vi "Characterise Polarisation.vi"() -> ()   [LabVIEW 2019]
panel:
  in  "Background Power (mW)":dbl format="%#_13g"
  in  "?":refnum<k7>(container)
  in  "Wavelength (nm)":dbl=400.0 caption="Wavelength (0.0)"
  in  "?":T1(tab)
  out "?":cluster{dbl[], dbl[]}[](graph)
  out "Current Scan Angle:":i32
  in  "Step Size:":i32=5
  in  "Full Rotation":bool
  in  "?":bool
  out "Stokes Vector:":dbl[](array[numeric]) format="%.3g"
  out "XY Graph 2":cluster{dbl[], dbl[]}[](graph)
  in  "?":refnum<k7>(container)
  out "Zero Angle on Stage :":dbl format="%#.1g"
  in  "?":enum32{"First Waveplate", "Second Waveplate"}(tab)
  out "XY Graph":cluster{dbl[], dbl[]}[](graph)
  out "?":cluster{dbl[], dbl[]}[](graph)
  out "?":cluster{dbl[], dbl[]}[](graph)
  out "Stokes Vector 2":dbl[](array[numeric]) format="%.3g"
  out "CPL 1:":dbl format="%#_4g"
  out "Stokes Vector":dbl[](array[numeric]) format="%.3g"
  out "CPL 2:":dbl format="%#.2g"
  in  "Full":bool
  in  "Step Size:":i32=10
  out "?":i32
  out "Current Scan Angle:":i32
  in  "?":bool
  in  "?":bool
  # "Polarisation Characterisation"
  # "This software uses the rotation of a quarter-wave plate and a power meter to characterise any given input laser polarisation. Specifically, it has been designed to produce and characterise right and left circulalry polarised light by using a motorised rotating waveplate.\n\nBefore use, please ensure:\n\n     - the power meter is turned on and connected to the PC/Laptop\n     using the mini-USB cable\n\n     - the motorised waveplate (if using) is connected to the \n     PC/Laptop using the USB 3.0 cable\n\n     - the laser beam is aimed at the power meter\n\n     - a polariser is placed in the beam path before the power meter\n\n     - the correct operating wavelength has been entered below\n     (the default is 400 nm)\n\nThen select the required function from the tab list, complete any further necessary steps and press 'Run' to execute the code."
  # "Half Rotation"
  # "This tab is used to calculate the Stoke's vector for any given input polarisation.\n\n     1. Choose to perform the measurment over a full or half rotation of the waveplate. The default is a full rotation.\n\n     2. Set the 'Step Size' for the quarter-wave plate. This must be an even divisor of 180. The default value is 10. \n\n     3. Insert the quarter-wave plate into the beam path before the polariser. Set the waveplate to zero degrees.\n\n     4. 'Run' the code.\n\n     5. Set the waveplate to the 'Current Scan Angle' and press 'Record' to save the power meter reading. Repeat this for all scan angles.\n\n     6. The scan will be displayed on the graph along with a fit using various sines and cosines (see paper for details). The Stokes vector will be displayed adjacent."
  # "This tab is used to produce pure circularly polarised light.\n\n     1. Set the perameters for the Stokes vector measurment.\n\n     2. 'Run' the code. This will find the two CPL angles on the waveplate.\n\n     3. Set the second waveplate to the 'Current Scan Angle' and press record. Repeat for poth angles.\n\n     4. The CPL angles and associated Stokes vectors are calculated and shown adjacent."
  # "Half"
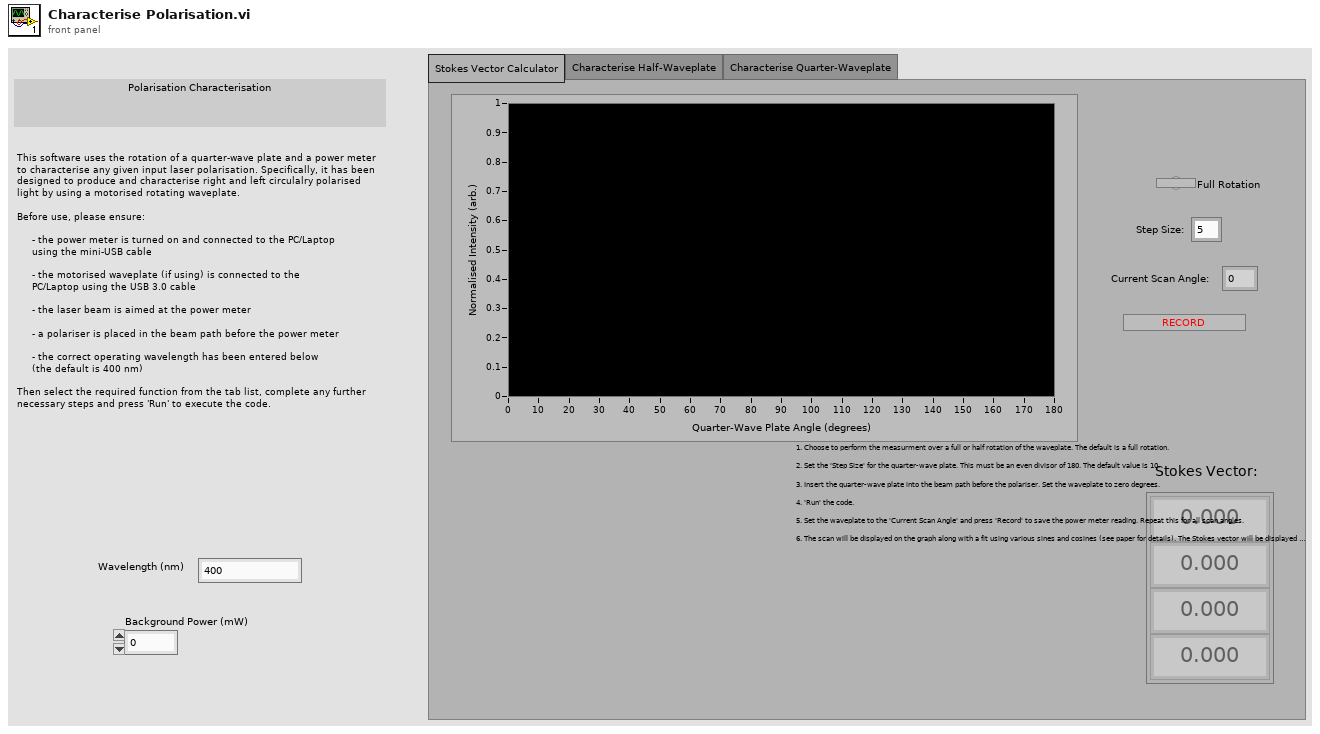
[diagram p1: front panel]
types:
  T1 = enum32{"Stokes Vector Calculator", "Characterise Half-Waveplate", "Characterise Quarter-Waveplate"}
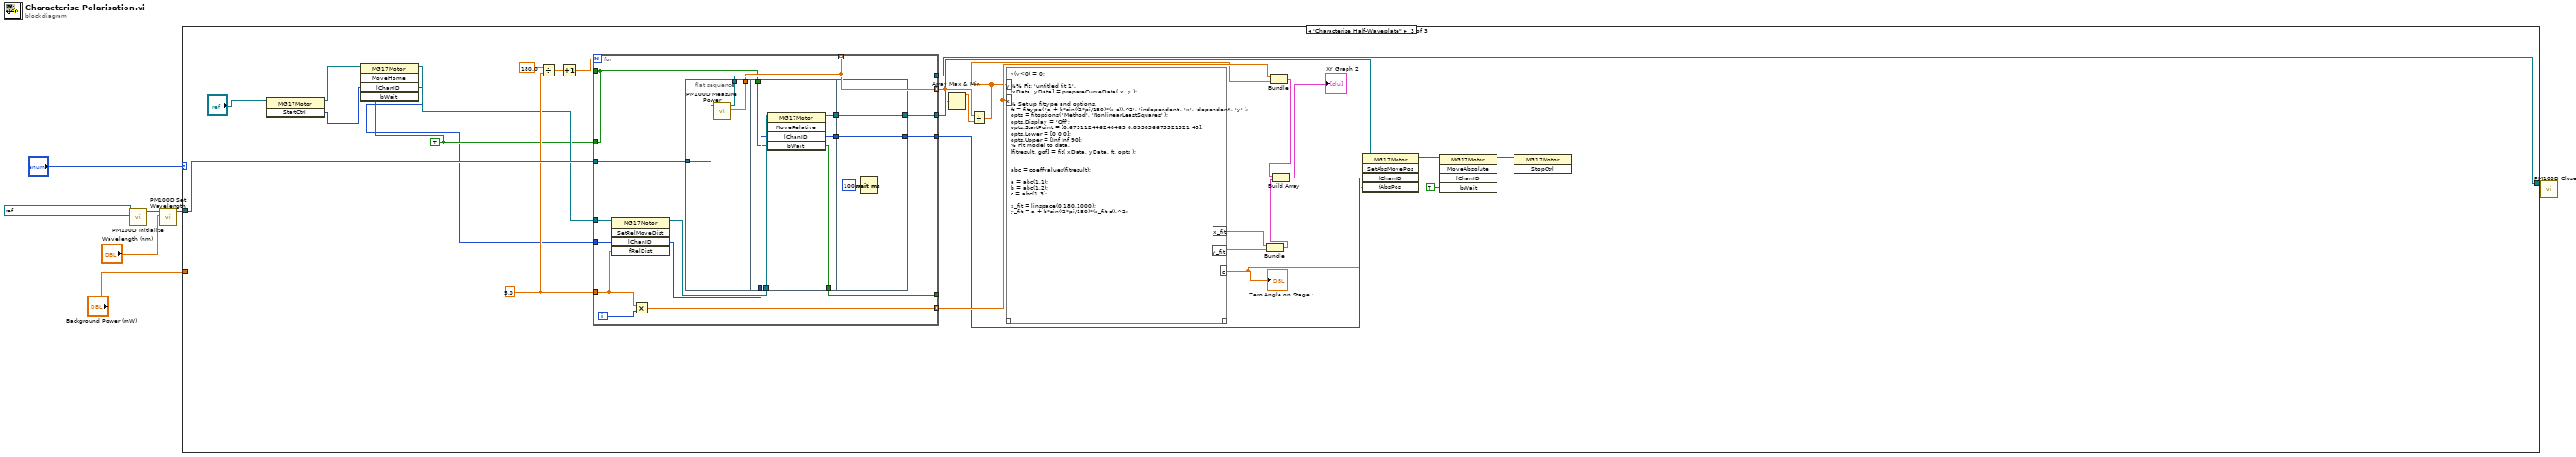
[diagram p0: block diagram]
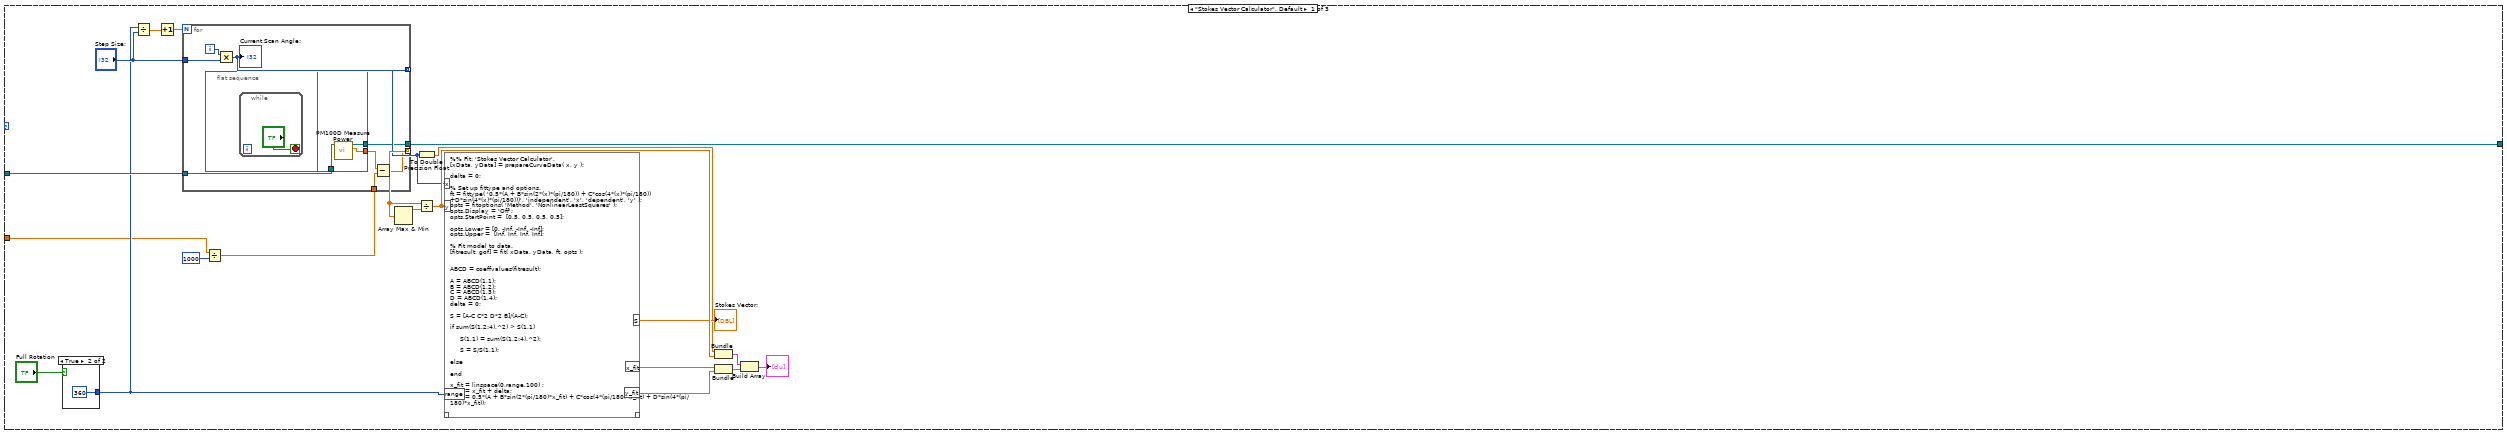
[diagram p2: hidden frame]
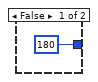
[diagram p3: hidden frame]
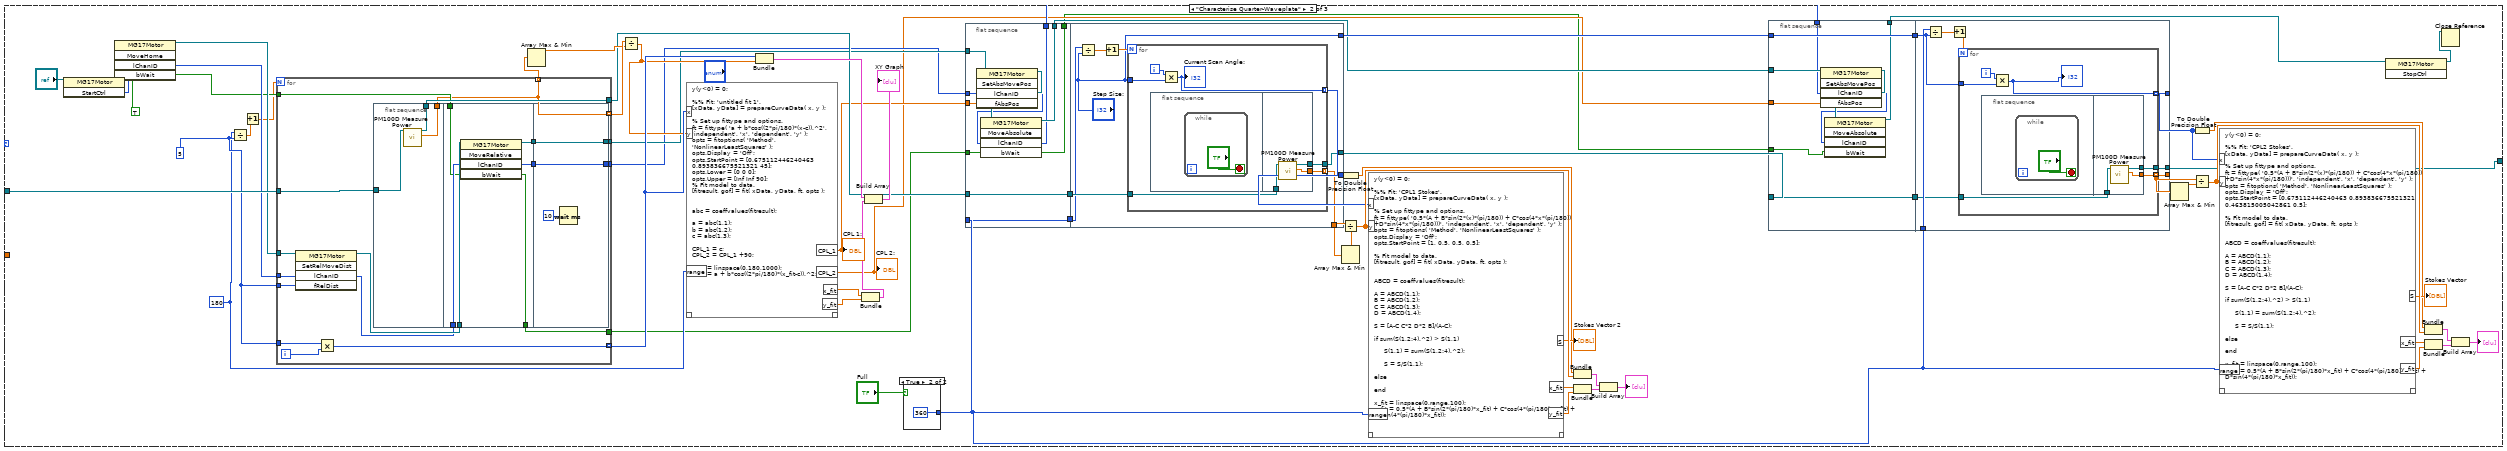
[diagram p4: hidden frame]
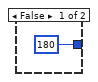
[diagram p5: hidden frame]
diagram:
  n1 = call <instrlib>:"PM100D Initialize.vi"("resource name"=refnum<visa-resource-name> "USB0::0x1313::0x8079::P1002885::INSTR") -> ("instrument handle out"=w6:refnum<visa-resource-name>)  [unwired: 9 in, 1 out]
  n2 = call <instrlib>:"PM100D Set Wavelength.vi"("Wavelength (0.0)"="Wavelength (nm)", "instrument handle"=w6) -> ("instrument handle out"=w3:refnum<visa-resource-name>)  [unwired: 8 in, 1 out]
  n3 = case shown="\"Characterise Half-Waveplate\"" "?" {
    tunnel: w3 -> [w25 w102 w220]
    tunnel: [w23 w57 w214] -> w2
    tunnel: "Background Power (mW)" -> [w10 _ _]
    frame "Stokes Vector Calculator", Default {
      n4 = case shown="True" "Full Rotation" {
        tunnel: [180 360] -> w11
        frame False {
        }
        frame True {
        }
      }
      n5 = Divide(x=w11, y="Step Size:") -> (x/y=w27:dbl)
      n6 = Increment(x=w27) -> (x+1=w26:dbl)
      n7 = Divide(x=w10, y=1000) -> (x/y=w8:dbl)
      n8 = for {
        N: w26 -> [_]
        tunnel: "Step Size:" -> [w35]
        tunnel: w25 -> [w36]
        tunnel: [w37] -> w14 mode=indexing
        tunnel: [w31] -> w22 mode=indexing
        tunnel: [w34] -> w23
        tunnel: w8 -> [w33]
        i -> [w38]
        n9 = flat-sequence {
          tunnel: w36 -> [w42]
          tunnel: [w41] -> w32
          tunnel: [w40] -> w34
          frame #0 {
            n10 = while {
              stop <- "?" stop-if-true
            }
          }
          frame #1 {
            n11 = call <instrlib>:"PM100D Measure Power.vi"("instrument handle"=w42) -> ("Power"=w41:dbl, "instrument handle out"=w40:refnum<visa-resource-name>)  [unwired: 8 in, 1 out]
          }
        }
        n12 = Multiply(x=w38, y=w35) -> (x*y=w37:i32)
        "Current Scan Angle:" <- w37
        n13 = Subtract(x=w32, y=w33) -> (x-y=w31:dbl)
      }
      n14 = Array Max & Min(array=w22) -> (max value=w21:dbl)  [unwired: 3 out]
      n15 = Divide(x=w22, y=w21) -> (x/y=w20:dbl[])
      n16 = To Double Precision Float(number=w14) -> (double precision float=w13:dbl[])
      n17 = script code="%% Fit: 'Stokes Vector Calculator'.\n[xData, yData] = prepareCurveData( x, y );\n\ndelta = 0;\n\n% Set up fittype and options.\nft = fittype( '0.5*(A + B*sin(2*(x)*(pi/180)) + C*cos(4*(x)*(pi/180)) +D*sin(4*(x)*(pi/180)))', 'independent', 'x', 'dependent', 'y' );\nopts = fitoptions( 'Method', 'NonlinearLeastSquares' );\nopts.Display = 'Off';\nopts.StartPoint =  [0.5, 0.5, 0.5, 0.5];\n\nopts.Lower = [0, -Inf, -Inf, -Inf];\nopts.Upper =  [Inf, Inf, Inf, Inf];\n\n% Fit model to data.\n[fitresult, gof] = fit( xData, yData, ft, opts );\n\n\nABCD = coeffvalues(fitresult);\n\nA = ABCD(1,1); \nB = ABCD(1,2);\nC = ABCD(1,3);\nD = ABCD(1,4);\ndelta = 0;\n\nS = [A-C C*2 D*2 B]/(A-C);\n\nif sum(S(1,2:4).^2) > S(1,1)\n\n     S(1,1) = sum(S(1,2:4).^2);\n\n     S = S/S(1,1);\n\nelse\n\nend\n\nx_fit = linspace(0,range,100) ;\nx_fit = x_fit + delta;\ny_fit = 0.5*(A + B*sin(2*(pi/180)*x_fit) + C*cos(4*(pi/180)*x_fit) + D*sin(4*(pi/180)*x_fit));"("x"=w14, "y"=w20, "range"=w11) -> ("S"=→"Stokes Vector:":dbl[], "x_fit"=w18:dbl[], "y_fit"=w17:dbl[])  [unwired: 1 in, 1 out]
      n18 = Bundle(w13, w20) -> (w16:cluster{dbl[], dbl[]})  [unwired: 1 in]
      n19 = Bundle(w18, w17) -> (w12:cluster{dbl[], dbl[]})  [unwired: 1 in]
      n20 = Build Array(w16, w12) -> (→"?":cluster{dbl[], dbl[]}[])
    }
    frame "Characterise Quarter-Waveplate" {
      w98 = 5 ("Step Size:")
      w89 = 180
      n21 = invoke class="MG17Motor" method="StartCtrl"(reference="?") -> (reference out=w105:refnum<k7>, "StartCtrl"=w103:i32)  [unwired: 2 in, 1 out]
      n22 = invoke class="MG17Motor" method="MoveHome"(reference=w105, "lChanID"=w103, "bWait"=TRUE) -> (reference out=w101:refnum<k7>, "lChanID"=w100:i32, "bWait"=w99:bool)  [unwired: 2 in, 2 out]
      n23 = Divide(x=w89, y=w98) -> (x/y=w97:dbl)
      n24 = Increment(x=w97) -> (x+1=w96:dbl)
      n25 = for {
        N: w96 -> [_]
        tunnel: w102 -> [w181]
        tunnel: w101 -> [w180]
        tunnel: w100 -> [w179]
        tunnel: w98 -> [w178]
        tunnel: [w177] -> w71
        tunnel: [w169] -> w87 mode=indexing
        tunnel: w99 -> [w174]
        tunnel: w98 -> [w172]
        tunnel: [w171] -> w95 mode=indexing
        tunnel: [w170] -> w53
        tunnel: [w169] -> w88 mode=indexing
        tunnel: [w168] -> w52
        tunnel: [w167] -> w50
        i -> [w173]
        n26 = invoke class="MG17Motor" method="SetRelMoveDist"(reference=w180, "lChanID"=w179, "fRelDist"=w178) -> (reference out=w176:refnum<k7>, "lChanID"=w175:i32)  [unwired: 2 in, 3 out]
        n27 = Multiply(x=w172, y=w173) -> (x*y=w171:i32)
        n28 = flat-sequence {
          tunnel: w181 -> [w184]
          tunnel: [w183] -> w177
          tunnel: [w182] -> w169
          tunnel: w176 -> [w190]
          tunnel: w175 -> [w189]
          tunnel: w174 -> [w188]
          tunnel: [w185] -> w167
          tunnel: [w187] -> w166
          tunnel: [w186] -> w165
          tunnel: [w192] -> w168
          tunnel: [w193] -> w170
          tunnel: w166 -> [w193]
          tunnel: w165 -> [w192]
          frame #0 {
            n29 = call <instrlib>:"PM100D Measure Power.vi"("instrument handle"=w184) -> ("Power"=w182:dbl, "instrument handle out"=w183:refnum<visa-resource-name>)  [unwired: 8 in, 1 out]
          }
          frame #1 {
            n30 = invoke class="MG17Motor" method="MoveRelative"(reference=w190, "lChanID"=w189, "bWait"=w188) -> (reference out=w187:refnum<k7>, "lChanID"=w186:i32, "bWait"=w185:bool)  [unwired: 2 in, 2 out]
          }
          frame #2 {
            n31 = Wait (ms)(milliseconds to wait=u32 10) -> ()  [unwired: 1 out]
          }
        }
      }
      n32 = Array Max & Min(array=w88) -> (max value=w86:dbl)  [unwired: 3 out]
      n33 = Divide(x=w87, y=w86) -> (x/y=w85:dbl[])
      n34 = script code="y(y<0) = 0;\n\n%% Fit: 'untitled fit 1'.\n[xData, yData] = prepareCurveData( x, y );\n\n% Set up fittype and options.\nft = fittype( 'a + b*cos((2*pi/180)*(x-c)).^2', 'independent', 'x', 'dependent', 'y' );\nopts = fitoptions( 'Method', 'NonlinearLeastSquares' );\nopts.Display = 'Off';\nopts.StartPoint = [0.675112446240463 0.893836675521321 45];\nopts.Lower = [0 0 0];\nopts.Upper = [Inf Inf 90]; \n% Fit model to data.\n[fitresult, gof] = fit( xData, yData, ft, opts );\n\n\nabc = coeffvalues(fitresult);\n\na = abc(1,1);\nb = abc(1,2);\nc = abc(1,3);\n\nCPL_1 = c;\nCPL_2 = CPL_1 +90;\n\nx_fit = linspace(0,180,1000);\ny_fit = a + b*cos((2*pi/180)*(x_fit-c)).^2;"("x"=w95, "y"=w85, "range"=w89) -> ("x_fit"=w94:dbl[], "y_fit"=w93:dbl[], "CPL_1"=w51:dbl, "CPL_2"=w45:dbl)  [unwired: 1 in, 1 out]
      "CPL 1:" <- w51
      "CPL 2:" <- w45
      n35 = Bundle(w95, w85) -> (w91:cluster{i32[], dbl[]})  [unwired: 1 in]
      n36 = Bundle(w94, w93) -> (w92:cluster{dbl[], dbl[]})  [unwired: 1 in]
      n37 = Build Array(w91, w92) -> (→"XY Graph":cluster{dbl[], dbl[]}[])
      n38 = case shown="True" "Full" {
        tunnel: [180 360] -> w59
        frame False {
        }
        frame True {
        }
      }
      n39 = flat-sequence {
        tunnel: w59 -> [w143]
        tunnel: w71 -> [w144]
        tunnel: [w144] -> w55
        tunnel: [w143] -> w54
        tunnel: w53 -> [w142]
        tunnel: w52 -> [w140]
        tunnel: w51 -> [w139]
        tunnel: w50 -> [w137]
        tunnel: [w136] -> w47
        tunnel: [w135] -> w46
        tunnel: [w134] -> w44
        tunnel: [w150] -> w82
        tunnel: [w149] -> w74
        tunnel: [w146] -> w58
        tunnel: ["Step Size:"] -> w56
        tunnel: w55 -> [w148]
        tunnel: w54 -> [w147]
        frame #0 {
          n40 = invoke class="MG17Motor" method="SetAbsMovePos"(reference=w142, "lChanID"=w140, "fAbsPos"=w139) -> (reference out=w141:refnum<k7>, "lChanID"=w138:i32)  [unwired: 2 in, 3 out]
          n41 = invoke class="MG17Motor" method="MoveAbsolute"(reference=w141, "lChanID"=w138, "bWait"=w137) -> (reference out=w136:refnum<k7>, "lChanID"=w135:i32, "bWait"=w134:bool)  [unwired: 2 in, 2 out]
        }
        frame #1 {
          n42 = Divide(x=w147, y="Step Size:") -> (x/y=w152:dbl)
          n43 = Increment(x=w152) -> (x+1=w151:dbl)
          n44 = for {
            N: w151 -> [_]
            tunnel: "Step Size:" -> [w154]
            tunnel: w148 -> [w156]
            tunnel: [w157] -> w149 mode=indexing
            tunnel: [w155] -> w150 mode=indexing
            tunnel: [w153] -> w146
            i -> [w158]
            n45 = flat-sequence {
              tunnel: w156 -> [w162]
              tunnel: [w161] -> w155
              tunnel: [w160] -> w153
              frame #0 {
                n46 = while {
                  stop <- "?" stop-if-true
                }
              }
              frame #1 {
                n47 = call <instrlib>:"PM100D Measure Power.vi"("instrument handle"=w162) -> ("Power"=w161:dbl, "instrument handle out"=w160:refnum<visa-resource-name>)  [unwired: 8 in, 1 out]
              }
            }
            n48 = Multiply(x=w158, y=w154) -> (x*y=w157:i32)
            "Current Scan Angle:" <- w157
          }
        }
      }
      n49 = Array Max & Min(array=w82) -> (max value=w81:dbl)  [unwired: 3 out]
      n50 = Divide(x=w82, y=w81) -> (x/y=w80:dbl[])
      n51 = To Double Precision Float(number=w74) -> (double precision float=w73:dbl[])
      n52 = script code="y(y<0) = 0;\n\n%% Fit: 'CPL1 Stokes'.\n[xData, yData] = prepareCurveData( x, y );\n\n% Set up fittype and options.\nft = fittype( '0.5*(A + B*sin(2*(x)*(pi/180)) + C*cos(4*x*(pi/180)) +D*sin(4*x*(pi/180)))', 'independent', 'x', 'dependent', 'y' );\nopts = fitoptions( 'Method', 'NonlinearLeastSquares' );\nopts.Display = 'Off';\nopts.StartPoint = [1, 0.5, 0.5, 0.5];\n\n% Fit model to data.\n[fitresult, gof] = fit( xData, yData, ft, opts );\n\n\nABCD = coeffvalues(fitresult);\n\nA = ABCD(1,1); \nB = ABCD(1,2);\nC = ABCD(1,3);\nD = ABCD(1,4);\n\nS = [A-C C*2 D*2 B]/(A-C);\n\nif sum(S(1,2:4).^2) > S(1,1)\n\n     S(1,1) = sum(S(1,2:4).^2);\n\n     S = S/S(1,1);\n\nelse\n\nend\n\nx_fit = linspace(0,range,100);\ny_fit = 0.5*(A + B*sin(2*(pi/180)*x_fit) + C*cos(4*(pi/180)*x_fit) + D*sin(4*(pi/180)*x_fit));"("x"=w74, "y"=w80, "range"=w59) -> ("S"=→"Stokes Vector 2":dbl[], "x_fit"=w78:dbl[], "y_fit"=w77:dbl[])  [unwired: 1 in, 1 out]
      n53 = Bundle(w73, w80) -> (w76:cluster{dbl[], dbl[]})  [unwired: 1 in]
      n54 = Bundle(w78, w77) -> (w72:cluster{dbl[], dbl[]})  [unwired: 1 in]
      n55 = Build Array(w76, w72) -> (→"?":cluster{dbl[], dbl[]}[])
      n56 = flat-sequence {
        tunnel: w56 -> [w114]
        tunnel: w58 -> [w115]
        tunnel: [w115] -> w49
        tunnel: [w114] -> w48
        tunnel: w47 -> [w111]
        tunnel: w46 -> [w110]
        tunnel: w45 -> [w109]
        tunnel: w44 -> [w108]
        tunnel: [w107] -> w43
        tunnel: [w121] -> w70
        tunnel: [w120] -> w62
        tunnel: w59 -> [w119]
        tunnel: [w117] -> w57
        tunnel: w49 -> [w118]
        tunnel: w48 -> [w116]
        frame #0 {
          n57 = invoke class="MG17Motor" method="SetAbsMovePos"(reference=w111, "lChanID"=w110, "fAbsPos"=w109) -> (reference out=w113:refnum<k7>, "lChanID"=w112:i32)  [unwired: 2 in, 3 out]
          n58 = invoke class="MG17Motor" method="MoveAbsolute"(reference=w113, "lChanID"=w112, "bWait"=w108) -> (reference out=w107:refnum<k7>)  [unwired: 2 in, 4 out]
        }
        frame #1 {
          n59 = Divide(x=w119, y=w116) -> (x/y=w123:dbl)
          n60 = Increment(x=w123) -> (x+1=w122:dbl)
          n61 = for {
            N: w122 -> [_]
            tunnel: w116 -> [w126]
            tunnel: w118 -> [w128]
            tunnel: [w124] -> w120 mode=indexing
            tunnel: [w127] -> w121 mode=indexing
            tunnel: [w125] -> w117
            i -> [w129]
            n62 = flat-sequence {
              tunnel: w128 -> [w133]
              tunnel: [w132] -> w127
              tunnel: [w131] -> w125
              frame #0 {
                n63 = while {
                  stop <- "?" stop-if-true
                }
              }
              frame #1 {
                n64 = call <instrlib>:"PM100D Measure Power.vi"("instrument handle"=w133) -> ("Power"=w132:dbl, "instrument handle out"=w131:refnum<visa-resource-name>)  [unwired: 8 in, 1 out]
              }
            }
            n65 = Multiply(x=w129, y=w126) -> (x*y=w124:i32)
            "?" <- w124
          }
        }
      }
      n66 = Array Max & Min(array=w70) -> (max value=w69:dbl)  [unwired: 3 out]
      n67 = Divide(x=w70, y=w69) -> (x/y=w68:dbl[])
      n68 = To Double Precision Float(number=w62) -> (double precision float=w61:dbl[])
      n69 = script code="y(y<0) = 0;\n\n%% Fit: 'CPL2 Stokes'.\n[xData, yData] = prepareCurveData( x, y );\n\n% Set up fittype and options.\nft = fittype( '0.5*(A + B*sin(2*(x)*(pi/180)) + C*cos(4*x*(pi/180)) +D*sin(4*x*(pi/180)))', 'independent', 'x', 'dependent', 'y' );\nopts = fitoptions( 'Method', 'NonlinearLeastSquares' );\nopts.Display = 'Off';\nopts.StartPoint = [0.675112446240463 0.893836675521321 0.463815005042861 0.5];\n\n% Fit model to data.\n[fitresult, gof] = fit( xData, yData, ft, opts );\n\n\nABCD = coeffvalues(fitresult);\n\nA = ABCD(1,1); \nB = ABCD(1,2);\nC = ABCD(1,3);\nD = ABCD(1,4);\n\nS = [A-C C*2 D*2 B]/(A-C);\n\nif sum(S(1,2:4).^2) > S(1,1)\n\n     S(1,1) = sum(S(1,2:4).^2);\n\n     S = S/S(1,1);\n\nelse\n\nend\n\nx_fit = linspace(0,range,100);\ny_fit = 0.5*(A + B*sin(2*(pi/180)*x_fit) + C*cos(4*(pi/180)*x_fit) + D*sin(4*(pi/180)*x_fit));"("x"=w62, "y"=w68, "range"=w59) -> ("S"=→"Stokes Vector":dbl[], "x_fit"=w66:dbl[], "y_fit"=w65:dbl[])  [unwired: 1 in, 1 out]
      n70 = invoke class="MG17Motor" method="StopCtrl"(reference=w43) -> (reference out=w84:refnum<k7>)  [unwired: 2 in, 2 out]
      n71 = Bundle(w61, w68) -> (w64:cluster{dbl[], dbl[]})  [unwired: 1 in]
      n72 = Bundle(w66, w65) -> (w60:cluster{dbl[], dbl[]})  [unwired: 1 in]
      n73 = Close Reference(reference=w84) -> ()  [unwired: 1 in, 1 out]
      n74 = Build Array(w64, w60) -> (→"?":cluster{dbl[], dbl[]}[])
    }
    frame "Characterise Half-Waveplate" {
      w195 = TRUE ("bWait")
      w219 = sgl 5.0 ("fRelDist")
      n75 = invoke class="MG17Motor" method="StartCtrl"(reference="?") -> (reference out=w198:refnum<k7>, "StartCtrl"=w197:i32)  [unwired: 2 in, 1 out]
      n76 = invoke class="MG17Motor" method="MoveHome"(reference=w198, "lChanID"=w197, "bWait"=w195) -> (reference out=w196:refnum<k7>, "lChanID"=w194:i32)  [unwired: 2 in, 3 out]
      n77 = Divide(x=sgl 180.0, y=w219) -> (x/y=w217:sgl)
      n78 = Increment(x=w217) -> (x+1=w216:sgl)
      n79 = for {
        N: w216 -> [_]
        tunnel: w220 -> [w237]
        tunnel: [w236] -> w214
        tunnel: [w230] -> w206 mode=indexing
        tunnel: [w225] -> _
        tunnel: [w232] -> w215 mode=indexing
        tunnel: [w231] -> w213
        tunnel: [w230] -> _ mode=indexing
        tunnel: [w229] -> w204
        tunnel: [w228] -> _
        tunnel: w195 -> [w225]
        tunnel: w194 -> [w224]
        tunnel: w196 -> [w223]
        tunnel: w219 -> [w222]
        i -> [w233]
        n80 = invoke class="MG17Motor" method="SetRelMoveDist"(reference=w223, "lChanID"=w224, "fRelDist"=w222) -> (reference out=w235:refnum<k7>, "lChanID"=w234:i32)  [unwired: 2 in, 3 out]
        n81 = Multiply(x=w222, y=w233) -> (x*y=w232:sgl)
        n82 = flat-sequence {
          tunnel: w237 -> [w240]
          tunnel: [w239] -> w236
          tunnel: [w238] -> w230
          tunnel: w235 -> [w246]
          tunnel: w234 -> [w245]
          tunnel: w225 -> [w244]
          tunnel: [w241] -> w228
          tunnel: [w243] -> w227
          tunnel: [w242] -> w226
          tunnel: [w248] -> w229
          tunnel: [w249] -> w231
          tunnel: w227 -> [w249]
          tunnel: w226 -> [w248]
          frame #0 {
            n83 = call <instrlib>:"PM100D Measure Power.vi"("instrument handle"=w240) -> ("Power"=w238:dbl, "instrument handle out"=w239:refnum<visa-resource-name>)  [unwired: 8 in, 1 out]
          }
          frame #1 {
            n84 = invoke class="MG17Motor" method="MoveRelative"(reference=w246, "lChanID"=w245, "bWait"=w244) -> (reference out=w243:refnum<k7>, "lChanID"=w242:i32, "bWait"=w241:bool)  [unwired: 2 in, 2 out]
          }
          frame #2 {
            n85 = Wait (ms)(milliseconds to wait=u32 100) -> ()  [unwired: 1 out]
          }
        }
      }
      n86 = Array Max & Min(array=w206) -> (max value=w205:dbl)  [unwired: 3 out]
      n87 = Divide(x=w206, y=w205) -> (x/y=w207:dbl[])
      n88 = script code="y(y<0) = 0;\n\n%% Fit: 'untitled fit 1'.\n[xData, yData] = prepareCurveData( x, y );\n\n% Set up fittype and options.\nft = fittype( 'a + b*sin((2*pi/180)*(x-c)).^2', 'independent', 'x', 'dependent', 'y' );\nopts = fitoptions( 'Method', 'NonlinearLeastSquares' );\nopts.Display = 'Off';\nopts.StartPoint = [0.675112446240463 0.893836675521321 45];\nopts.Lower = [0 0 0];\nopts.Upper = [Inf Inf 90]; \n% Fit model to data.\n[fitresult, gof] = fit( xData, yData, ft, opts );\n\n\nabc = coeffvalues(fitresult);\n\na = abc(1,1);\nb = abc(1,2);\nc = abc(1,3);\n\nx_fit = linspace(0,180,1000);\ny_fit = a + b*sin((2*pi/180)*(x_fit-c)).^2;"("y"=w207, "x"=w215) -> ("x_fit"=w212:dbl[], "y_fit"=w211:dbl[], "c"=w203:dbl)  [unwired: 1 in, 1 out]
      "Zero Angle on Stage :" <- w203
      n89 = Bundle(w212, w211) -> (w208:cluster{dbl[], dbl[]})  [unwired: 1 in]
      n90 = Bundle(w215, w207) -> (w209:cluster{sgl[], dbl[]})  [unwired: 1 in]
      n91 = Build Array(w209, w208) -> (→"XY Graph 2":cluster{dbl[], dbl[]}[])
      n92 = invoke class="MG17Motor" method="SetAbsMovePos"(reference=w213, "lChanID"=w204, "fAbsPos"=w203) -> (reference out=w202:refnum<k7>, "lChanID"=w201:i32)  [unwired: 2 in, 3 out]
      n93 = invoke class="MG17Motor" method="MoveAbsolute"(reference=w202, "lChanID"=w201, "bWait"=TRUE) -> (reference out=w199:refnum<k7>)  [unwired: 2 in, 4 out]
      n94 = invoke class="MG17Motor" method="StopCtrl"(reference=w199) -> ()  [unwired: 2 in, 3 out]
    }
  }
  n95 = call <instrlib>:"PM100D Close.vi"("instrument handle"=w2) -> ()  [unwired: 10 in, 1 out]
